vi "alignRight.vi"(6 "useControlBodyOnly":bool, 8 "error in (no error)":errorcluster, 11 "refs":refnum<vi>[](array[refnum])) -> (0 "error out":errorcluster, 3 "refs(dup)":refnum<vi>[](array[refnum]))   [LabVIEW 2023]
doc: "Aligns all controls to the rightmost position among the input controls.\nThe rightmost coordinate is computed and applied to all controls."
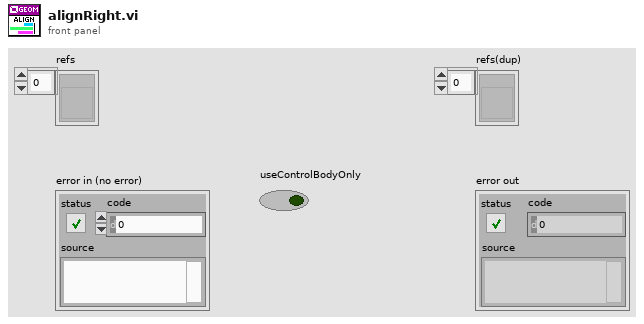
[diagram p1: front panel]
types:
  T1 = cluster{"left":i32, "top":i32, "right":i32, "bottom":i32}
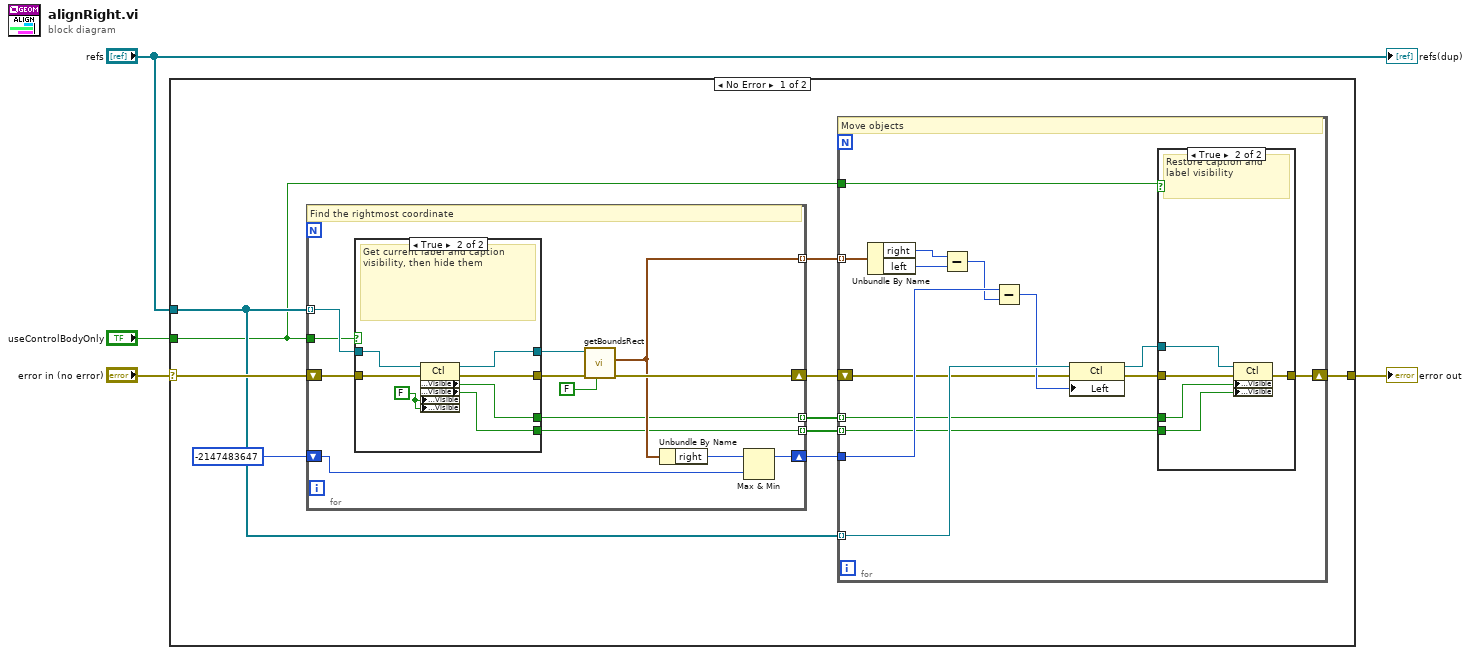
[diagram p0: block diagram]
diagram:
  n1 = case shown="No Error" "error in (no error)" {
    selector: "error in (no error)" -> [w14 w57]
    tunnel: [w11 w57] -> w3
    tunnel: "refs" -> [w12 _]
    tunnel: "useControlBodyOnly" -> [w7 _]
    frame No Error {
      n2 = for {
        tunnel: w12 -> [w41] mode=indexing
        shift-right: [w47] -> w10
        shift-left: w14 -> [w40]
        shift-right: [w44] -> w9
        shift-left: -2147483647 -> [w45]
        tunnel: [w43] -> w8 mode=indexing
        tunnel: w7 -> [w38]
        tunnel: [w37] -> w6 mode=indexing
        tunnel: [w36] -> w5 mode=indexing
        # "Find the rightmost coordinate"
        n3 = case shown="True" w38 {
          tunnel: [w49 w56] -> w42
          tunnel: w41 -> [w49 w55]
          tunnel: w40 -> [w48 w54]
          tunnel: [w48 w53] -> w39
          tunnel: [_ w52] -> w37
          tunnel: [_ w51] -> w36
          frame False {
            # "Do nothing"
          }
          frame True {
            w50 = FALSE ("Caption.Visible")
            # "Get current label and caption visibility, then hide them"
            n4 = property class="Ctl"(reference=w55, error in=w54, "Caption.Visible"=w50, "Label.Visible"=w50) -> (reference out=w56:refnum<vi>, error out=w53:errorcluster, "Caption.Visible"=w52:bool, "Label.Visible"=w51:bool)
          }
        }
        n5 = call "getBoundsRect.vi"("useControlBodyOnly"=FALSE ("ignoreCaption&Labels"), "error in (no error)"=w39, "ref"=w42) -> ("error out"=w47:errorcluster, "rect"=w43:T1)  [unwired: 6 in, 1 out]
        n6 = Unbundle By Name(w43) -> ("right"=w46:i32)
        n7 = Max & Min(x=w46, y=w45) -> (max(x,y)=w44:i32)  [unwired: 1 out]
      }
      n8 = for {
        tunnel: w12 -> [w28] mode=indexing
        shift-right: [w20] -> w11
        shift-left: w10 -> [w21]
        tunnel: w9 -> [w24]
        tunnel: w8 -> [w27] mode=indexing
        tunnel: w7 -> [w18]
        tunnel: w6 -> [w16] mode=indexing
        tunnel: w5 -> [w15] mode=indexing
        # "Move objects"
        n9 = Unbundle By Name(w27) -> ("right"=w26:i32, "left"=w25:i32)
        n10 = Subtract(x=w26, y=w25) -> (x-y=w23:i32)
        n11 = Subtract(x=w24, y=w23) -> (x-y=w22:i32)
        n12 = property class="Ctl"(reference=w28, error in=w21, "Left"=w22) -> (reference out=w17:refnum<vi>, error out=w19:errorcluster)
        n13 = case shown="True" w18 {
          tunnel: w17 -> [_ w34]
          tunnel: w19 -> [w29 w33]
          tunnel: [w29 w32] -> w20
          tunnel: w16 -> [_ w31]
          tunnel: w15 -> [_ w30]
          frame False {
            # "Do nothing"
          }
          frame True {
            # "Restore caption and label visibility"
            n14 = property class="Ctl"(reference=w34, error in=w33, "Caption.Visible"=w31, "Label.Visible"=w30) -> (error out=w32:errorcluster)  [unwired: 1 out]
          }
        }
      }
    }
    frame Error {
    }
  }
  "error out" <- w3
  "refs(dup)" <- "refs"
